vi "drawCircle.vi"(0 "reference":refnum<class "Graphics.lvclass">, 1 "rectangle":T1 {"height" format="%.2f"; "width" format="%.2f"; "y" format="%.2f"; "x" format="%.2f"}, 2 "lineWidth(1)":dbl=1.0 format="%.2f", 3 "color(if not used=default color)":u32=33554432 format="%.0x", 4 "fill?(F)":bool, 5 "error in (no error)":errorcluster) -> (14 "reference out":refnum<class "Graphics.lvclass">, 19 "error out":errorcluster)   [LabVIEW 2012, in "Graphics.lvclass"]
doc: "Draws a oval/circle"
uses:
  <resource>/Framework/Providers/Open_GDS/UML/Graphics_class/Graphics.lvclass
  <resource>/Framework/Providers/Open_GDS/UML/General/Rectangle/Rectangle Rectangle2D.ctl
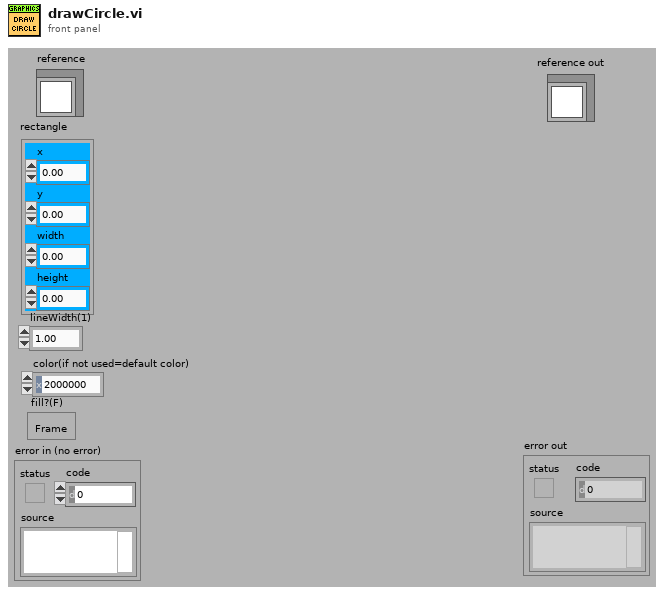
[diagram p1: front panel]
types:
  T1 = typedef "Rectangle Rectangle2D.ctl" = cluster{"x":dbl, "y":dbl, "width":dbl, "height":dbl}
  T2 = typedef "Graphics.lvclass/ObjectAttributes.ctl" = cluster{"drawColor":u32, "backgroundColor":u32, "font":T3, "fontType":T4, "picture":picture, "stroke":T5, "scaleX":dbl, "scaleY":dbl, "screenRef":refnum<vi>, "offsetX":dbl, "offsetY":dbl}
  T3 = typedef "Graphics.lvclass/FontType.ctl" = cluster{"Font Name:":string, "Size":i16, "Strikeout?":bool, "Italic?":bool, "Underline?":bool, "Outline?":bool, "Shadow?":bool, "Bold?":bool}
  T4 = typedef "Graphics.lvclass/LvFontType.ctl" = enum16{"User-specified Font", "Application Font", "System Font", "Dialog Font"}
  T5 = typedef "Graphics.lvclass/StrokeType.ctl" = enum16{"USE_DEFAULT", "SOLID", "DOTTED"}
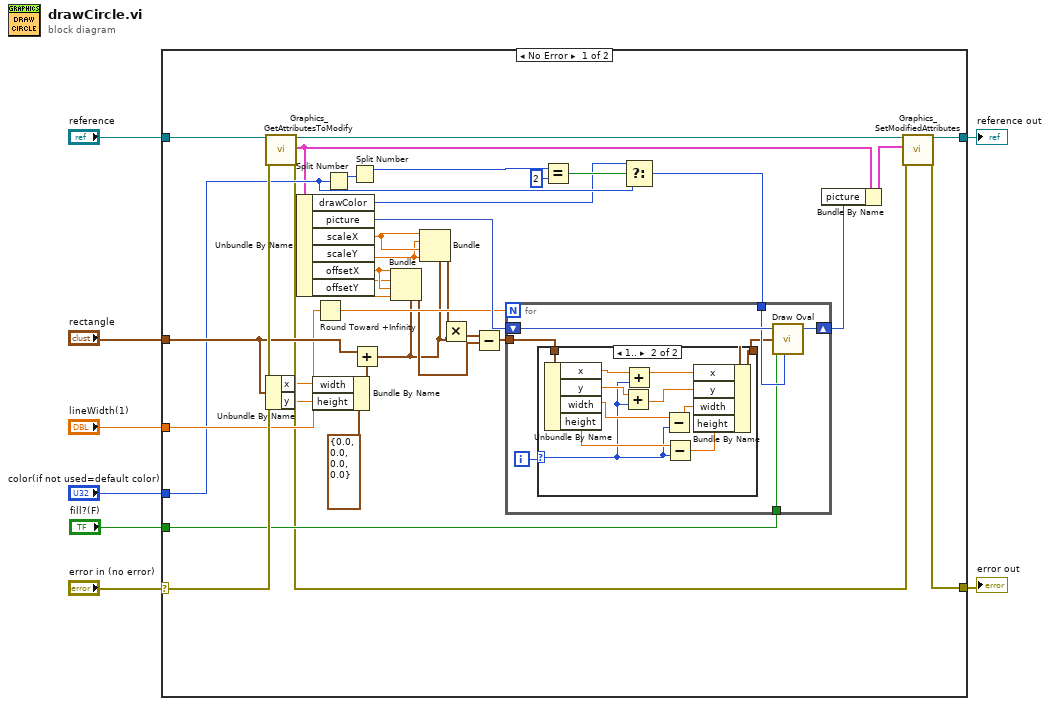
[diagram p0: block diagram]
diagram:
  n1 = case shown="No Error" "error in (no error)" {
    selector: "error in (no error)" -> [w39 w62]
    tunnel: "reference" -> [w42 w63]
    tunnel: [w41 w62] -> w7
    tunnel: [w40 w63] -> w6
    tunnel: "rectangle" -> [w38 _]
    tunnel: "lineWidth(1)" -> [w37 _]
    tunnel: "color(if not used=default color)" -> [w36 _]
    tunnel: "fill?(F)" -> [w35 _]
    frame No Error {
      n2 = call <resource>:"Graphics_GetAttributesToModify.vi"("reference in"=w42, "error in (no error)"=w39) -> ("reference out"=w34:refnum<class "Graphics.lvclass">, "Attributes"=w32:T2, "error out"=w33:errorcluster)  [unwired: 1 in, 14 out]
      n3 = Unbundle By Name(w38) -> ("x"=w17:dbl, "y"=w16:dbl)
      n4 = Unbundle By Name(w32) -> ("drawColor"=w23:u32, "picture"=w30:picture, "scaleX"=w20:dbl, "scaleY"=w19:dbl, "offsetX"=w12:dbl, "offsetY"=w11:dbl)
      n5 = Bundle By Name(cluster=T1 {"x"=0.0, "y"=0.0, "width"=0.0, "height"=0.0} ("x"), "width"=w17, "height"=w16) -> (w15:T1)
      n6 = Round Toward +Infinity(x=w37) -> (ceil(x): smallest int >= x=w29:dbl)
      n7 = Split Number(x=w36) -> (hi(x)=w27:u16)  [unwired: 1 out]
      n8 = Split Number(x=w27) -> (hi(x)=w26:u8)  [unwired: 1 out]
      n9 = Add(x=w38, y=w15) -> (x+y=w9:T1)
      n10 = Bundle(cluster=w9, "x"=w12, "y"=w11, "width"=w12, "height"=w11) -> (w10:T1)
      n11 = Bundle(cluster=w9, "x"=w20, "y"=w19, "width"=w20, "height"=w19) -> (w21:T1)
      n12 = Multiply(x=w21, y=w9) -> (x*y=w14:T1)
      n13 = Subtract(x=w14, y=w10) -> (x-y=w13:T1)
      n14 = Equal?(x=w26, y=u8 2) -> (x = y?=w24:bool)
      n15 = Select(t=w23, s=w24, f=w36) -> (s? t:f=w22:u32)
      n16 = for {
        N: w29 -> [_]
        tunnel: w13 -> [w45]
        tunnel: w22 -> [w48]
        shift-right: [w47] -> w28
        shift-left: w30 -> [w49]
        tunnel: w35 -> [w43]
        i -> [w44]
        n17 = case shown="1.." w44 {
          selector: w44 -> [_ w51]
          tunnel: [w50 w53] -> w46
          tunnel: w45 -> [w50 w52]
          frame 0, Default {
          }
          frame 1.. {
            n18 = Unbundle By Name(w52) -> ("x"=w61:dbl, "y"=w60:dbl, "width"=w59:dbl, "height"=w58:dbl)
            n19 = Add(x=w60, y=w51) -> (x+y=w56:dbl)
            n20 = Add(x=w61, y=w51) -> (x+y=w57:dbl)
            n21 = Subtract(x=w59, y=w51) -> (x-y=w55:dbl)
            n22 = Subtract(x=w58, y=w51) -> (x-y=w54:dbl)
            n23 = Bundle By Name(cluster=w52, "x"=w57, "y"=w56, "width"=w55, "height"=w54) -> (w53:T1)
          }
        }
        n24 = call <vilib>:"Draw Oval.vi"("picture"=w49, "rect"=w46, "fill?(F)"=w43, "color(black)"=w48) -> ("new picture"=w47:picture)  [unwired: 1 in, 4 out]
      }
      n25 = Bundle By Name(cluster=w32, "picture"=w28) -> (w31:T2)
      n26 = call <resource>:"Graphics_SetModifiedAttributes.vi"("reference in"=w34, "Attributes"=w31, "error in (no error)"=w33) -> ("reference out"=w40:refnum<class "Graphics.lvclass">, "error out"=w41:errorcluster)  [unwired: 3 in, 12 out]
    }
    frame Error {
    }
  }
  "reference out" <- w6
  "error out" <- w7
